vi "filter and get control value.vi"(8 "error in (no error)":errorcluster, 10 "Control label":string, 11 "VI (Caller)":refnum<vi>) -> (0 "error out":errorcluster, 3 "Value":string)   [LabVIEW 2020, in "ui-testing.lvlib"]
uses:
  ui-testing.lvlib
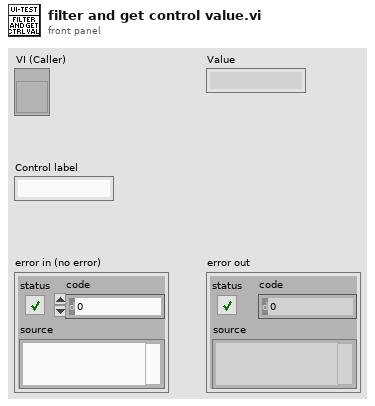
[diagram p1: front panel]
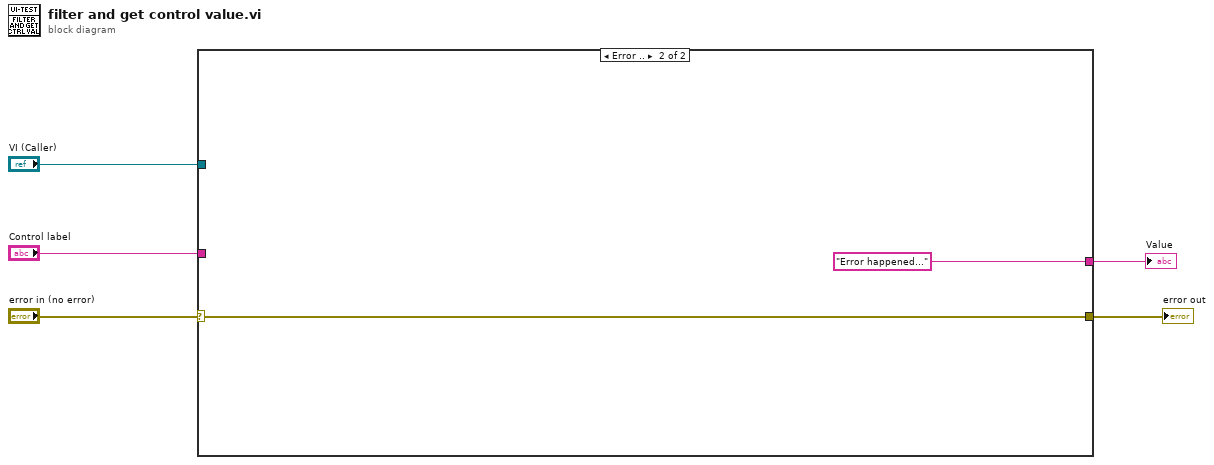
[diagram p0: block diagram]
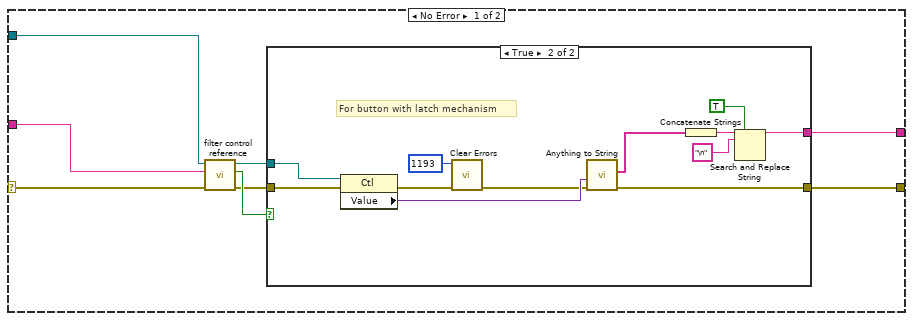
[diagram p2: hidden frame]
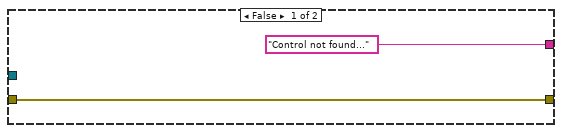
[diagram p3: hidden frame]
diagram:
  n1 = case shown="Error .." "error in (no error)" {
    selector: "error in (no error)" -> [w10 w29]
    tunnel: "Control label" -> [w9 _]
    tunnel: "VI (Caller)" -> [w8 _]
    tunnel: [w7 "Error happened..."] -> w2
    tunnel: [w6 w29] -> w1
    frame No Error {
      n2 = call "filter control reference.vi"("error in (no error)"=w10, "Control label"=w9, "VI (Caller)"=w8) -> ("error out"=w12:errorcluster, "Control found"=w13:bool, "Control ref"=w11:refnum<vi>)  [unwired: 6 in]
      n3 = case shown="True" w13 {
        tunnel: w12 -> [w15 w27]
        tunnel: w11 -> [_ w26]
        tunnel: ["Control not found..." w16] -> w7
        tunnel: [w15 w21] -> w6
        frame False {
        }
        frame True {
          # "For button with latch mechanism"
          n4 = property class="Ctl"(reference=w26, error in=w27) -> (error out=w24:errorcluster, "Value"=w25:variant)  [unwired: 1 out]
          n5 = call <vilib>:"Clear Errors.vi"("error in (no error)"=w24, "specific error code to clear (0: all)"=1193) -> ("error out"=w22:errorcluster)  [unwired: 4 in, 1 out]
          n6 = call <userlib>:"Anything to String.vi"("Error In"=w22, "Anything"=w25) -> ("Error Out"=w21:errorcluster, "Strings[]"=w17:string[])  [unwired: 7 in, 1 out]
          n7 = Concatenate Strings(w17) -> (w20:string)
          n8 = Search and Replace String(replace all?=TRUE ("replace all? (F)"), input string=w20, search string="\n") -> (result string=w16:string)  [unwired: 5 in, 3 out]
        }
      }
    }
    frame Error {
    }
  }
  "error out" <- w1
  "Value" <- w2
